vi "Color Sensor V3 CIE XYZ to sRGB.vi"(11 "CIE XYZ":cluster{"X":dbl, "Y":dbl, "Z":dbl}) -> (2 "sRGB Color":u32(colorbox), 3 "sRGB":cluster{"R":dbl, "G":dbl, "B":dbl})   [LabVIEW 2023]
uses:
  <vilib>/Analysis/Matrix/Datatypes/RealMatrix.ctl
  <vilib>/Analysis/baseanly.llb/Real A x B.vi
  <vilib>/Analysis/Matrix/NI_Matrix.lvlib
  <vilib>/Analysis/NI_AALBase.lvlib
panel:
  out "A x B":T1
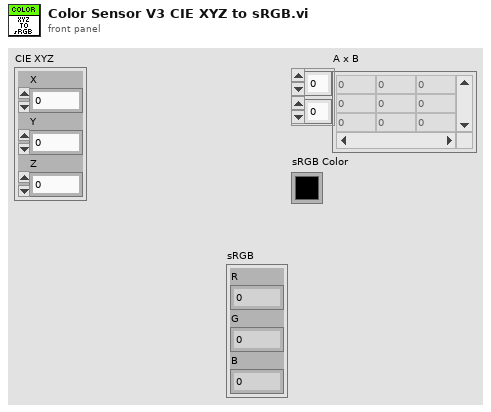
[diagram p1: front panel]
types:
  T1 = typedef "NI_Matrix.lvlib/RealMatrix.ctl" = dbl[][]
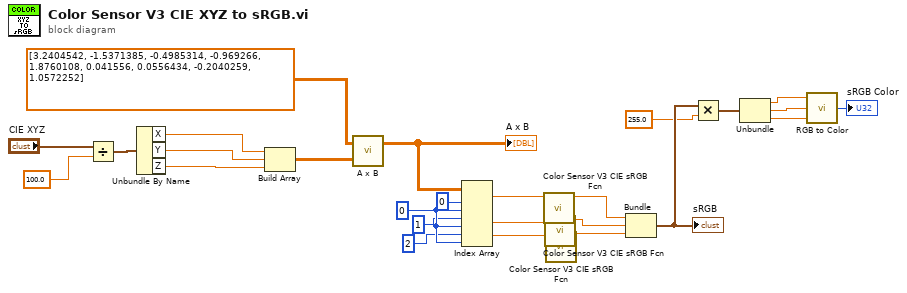
[diagram p0: block diagram]
diagram:
  w20 = 0 ("disabled index (col)")
  n1 = Divide(x="CIE XYZ", y=100.0) -> (x/y=w14:cluster{"X":dbl, "Y":dbl, "Z":dbl})
  n2 = Unbundle By Name(w14) -> ("X"=w26:dbl, "Y"=w25:dbl, "Z"=w24:dbl)
  n3 = Build Array(w26, w25, w24) -> (w23:T1)
  n4 = call-poly <vilib>:"A x B.vi"("B"=w23, "A"=T1 [[3.2404542, -1.5371385, -0.4985314], [-0.969266, 1.8760108, 0.041556], [0.0556434, -0.2040259, 1.0572252]] ("appended array")) -> ("A x B"=w21:T1)  [unwired: 1 out]
  "A x B" <- w21
  n5 = Index Array(array=w21, index (row) #1=0 ("disabled index (col)"), index (col) #1=w20, index (row) #2=1 ("disabled index (col)"), index (col) #2=w20, index (row) #3=2 ("disabled index (col)"), index (col) #3=w20) -> (element #1=w13:dbl, element #2=w11:dbl, element #3=w8:dbl)
  n6 = call "Color Sensor V3 CIE sRGB Fcn.vi"("Real Matrix Element"=w13) -> ("y"=w12:dbl)  [unwired: 10 in]
  n7 = call "Color Sensor V3 CIE sRGB Fcn.vi"("Real Matrix Element"=w11) -> ("y"=w10:dbl)  [unwired: 10 in]
  n8 = call "Color Sensor V3 CIE sRGB Fcn.vi"("Real Matrix Element"=w8) -> ("y"=w9:dbl)  [unwired: 10 in]
  n9 = Bundle("y"=w12, "y"=w10, "y"=w9) -> (w7:cluster{"y":dbl, "y":dbl, "y":dbl})  [unwired: 1 in]
  "sRGB" <- w7
  n10 = Multiply(x=w7, y=255.0) -> (x*y=w5:cluster{"y":dbl, "y":dbl, "y":dbl})
  n11 = Unbundle(w5) -> ("y"=w4:dbl, "y"=w3:dbl, "y"=w2:dbl)
  n12 = call <vilib>:"RGB to Color.vi"("B"=w2, "G"=w3, "R"=w4) -> ("Color"=→"sRGB Color":u32)
